vi "Configure Math (Base).vi"(0 "VISA resource name":refnum<visa-resource-name>, 5 "Mode":T1(ring), 11 "error in (no error)":errorcluster) -> (4 "VISA resource name out":refnum<visa-resource-name>, 15 "error out":errorcluster)   [LabVIEW 2015, in "ZhiYuan ZDS Series for TCP.lvlib"]
doc: "Configures the setting for advanced math operation."
uses:
  ZhiYuan ZDS Series for TCP.lvlib
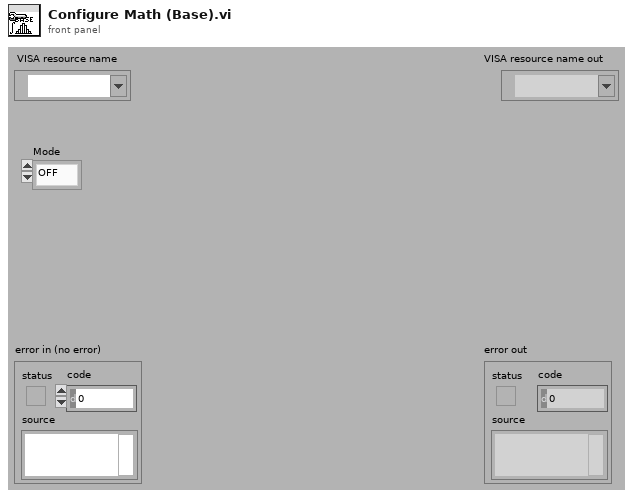
[diagram p1: front panel]
types:
  T1 = enum16{"OFF", "Add", "Sub", "Mul", "Div", "Differential", "Integral", "FFT", "Filter"}
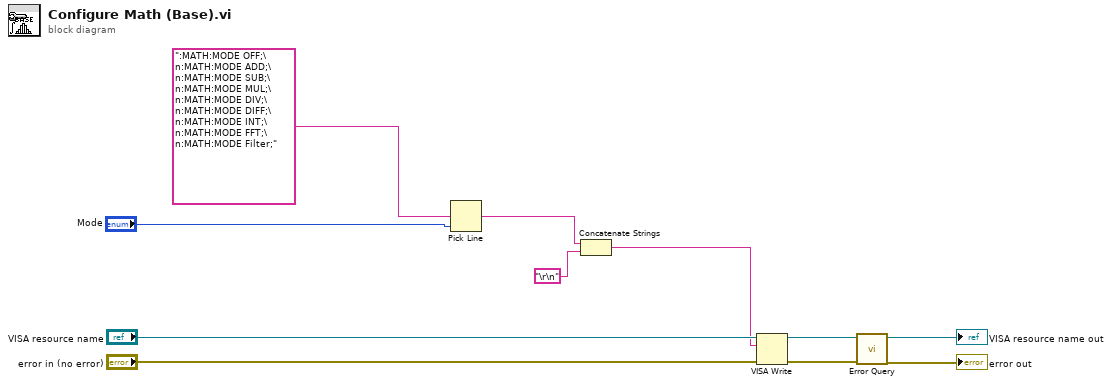
[diagram p0: block diagram]
diagram:
  n1 = Pick Line(multi-line string=":MATH:MODE OFF;\n:MATH:MODE ADD;\n:MATH:MODE SUB;\n:MATH:MODE MUL;\n:MATH:MODE DIV;\n:MATH:MODE DIFF;\n:MATH:MODE INT;\n:MATH:MODE FFT;\n:MATH:MODE Filter;", line index="Mode") -> (output string=w3:string)  [unwired: 1 in]
  n2 = Concatenate Strings(w3, "\r\n") -> (w1:string)
  n3 = VISA Write(VISA resource name="VISA resource name", write buffer=w1, error in (no error)="error in (no error)") -> (VISA resource name out=w9:refnum<visa-resource-name>, error out=w8:errorcluster)  [unwired: 1 out]
  n4 = call "Error Query.vi"("error in (no error)"=w8, "VISA resource name"=w9) -> ("error out"=→"error out":errorcluster, "VISA resource name out"=→"VISA resource name out":refnum<visa-resource-name>)  [unwired: 6 in, 2 out]
